vi "TDMS Write Group Data.vi"(8 "error in (no error)":errorcluster, 9 "Fields Array":T1[](array[typedef]), 10 "Channel Group":string, 11 "TDMS File Ref":refnum<k34>) -> (0 "error out":errorcluster, 3 "TDMS File Ref":refnum<k34>, 4 "Execution Time (ms)":u32)   [LabVIEW 2011]
uses:
  database/Fields/Field Record.ctl
  database/Fields/Field DataTypes.ctl
  database/Fields/Field NextItem.ctl
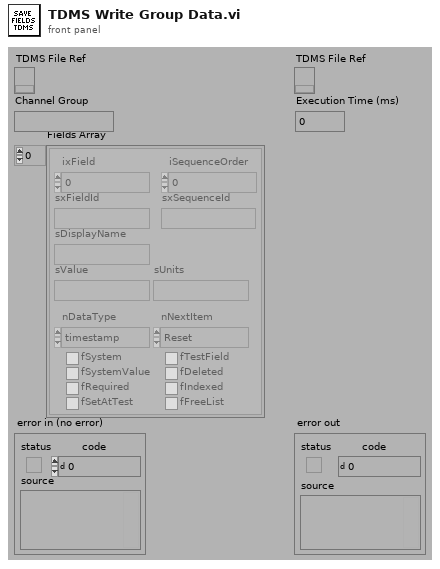
[diagram p1: front panel]
types:
  T1 = typedef "Field Record.ctl" = cluster{"ixField":i32, "iSequenceOrder":i32, "sxFieldId":string, "sxSequenceId":string, "sDisplayName":string, "sValue":string, "sUnits":string, "nDataType":T2, "nNextItem":T3, "fSystem":bool, "fSystemValue":bool, "fRequired":bool, "fSetAtTest":bool, "fTestField":bool, "fDeleted":bool, "fIndexed":bool, "fFreeList":bool}
  T2 = typedef "Field DataTypes.ctl" = enum32{"text", "numeric", "list", "timestamp", "boolean"}
  T3 = typedef "Field NextItem.ctl" = enum32{"Reset", "Retain", "Auto-Increment"}
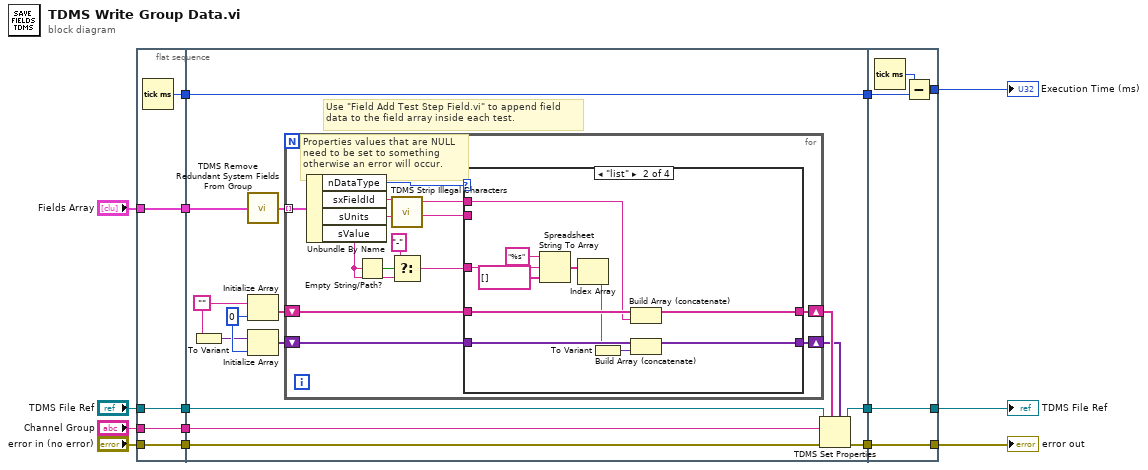
[diagram p0: block diagram]
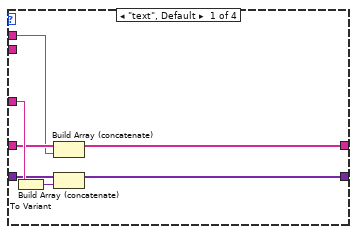
[diagram p2: hidden frame]
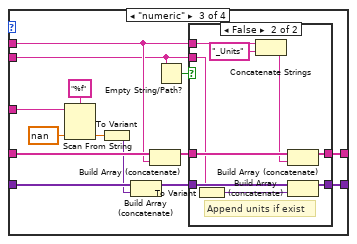
[diagram p3: hidden frame]
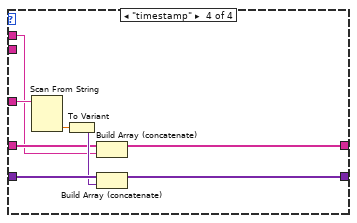
[diagram p5: hidden frame]
diagram:
  n1 = flat-sequence {
    tunnel: "Channel Group" -> [w17]
    tunnel: "error in (no error)" -> [w18]
    tunnel: "TDMS File Ref" -> [w19]
    tunnel: "Fields Array" -> [w20]
    tunnel: [w20] -> w7
    tunnel: [w19] -> w6
    tunnel: [w18] -> w5
    tunnel: [w17] -> w4
    tunnel: [w16] -> w2
    tunnel: [w30] -> w9
    tunnel: [w33] -> w8
    tunnel: w7 -> [w22]
    tunnel: w6 -> [w35]
    tunnel: w5 -> [w34]
    tunnel: w4 -> [w32]
    tunnel: [w31] -> w3
    tunnel: w2 -> [w31]
    tunnel: [w103] -> w11
    tunnel: [w104] -> w14
    tunnel: w9 -> [w104]
    tunnel: w8 -> [w103]
    tunnel: w3 -> [w101]
    tunnel: [w100] -> w1
    frame #0 {
      n2 = Tick Count (ms)() -> (millisecond timer value=w16:u32)
    }
    frame #1 {
      w27 = 0 ("dimension size")
      w23 = ""
      # "Use \"Field Add Test Step Field.vi\" to append field\ndata to the field array inside each test."
      n3 = To Variant(anything=w23) -> (Variant=w26:variant)
      n4 = call "TDMS Remove Redundant System Fields From Group.vi"("Fields In"=w22) -> ("Fields Out"=w21:T1[])
      n5 = Initialize Array(w23, w27) -> (w29:string[])
      n6 = Initialize Array(w26, w27) -> (w28:variant[])
      n7 = for {
        tunnel: w21 -> [w48] mode=indexing
        shift-right: [w40] -> w25
        shift-left: w29 -> [w42]
        shift-right: [w41] -> w24
        shift-left: w28 -> [w43]
        # "Properties values that are NULL\nneed to be set to something\notherwise an error will occur."
        n8 = Unbundle By Name(w48) -> ("nDataType"=w38:T2, "sxFieldId"=w44:string, "sUnits"=w36:string, "sValue"=w37:string)
        n9 = Empty String/Path?(string/path=w37) -> (empty?=w47:bool)
        n10 = call "TDMS Strip Illegal Characters.vi"("String"=w44) -> ("Legal String"=w39:string)  [unwired: 4 out]
        n11 = Select(t="-", s=w47, f=w37) -> (s? t:f=w46:string)
        n12 = case shown="\"numeric\"" w38 {
          tunnel: w46 -> [w55 w60 w75 w98]
          tunnel: w43 -> [w52 w64 w79 w97]
          tunnel: w42 -> [w54 w66 w80 w94]
          tunnel: [w49 w61 w70 w95] -> w41
          tunnel: [w53 w65 w71 w93] -> w40
          tunnel: w39 -> [w50 w62 w69 w92]
          tunnel: w36 -> [_ _ w67 _]
          frame "text", Default {
            n13 = To Variant(anything=w55) -> (Variant=w51:variant)
            n14 = Build Array (concatenate)(w54, w50) -> (w53:string[])
            n15 = Build Array (concatenate)(w52, w51) -> (w49:variant[])
          }
          frame "list" {
            n16 = Spreadsheet String To Array(format string="%s" ("delimiter (Tab)"), spreadsheet string=w60, array type (2D Dbl)=string[] []) -> (array=w58:string[])  [unwired: 1 in]
            n17 = Index Array(array=w58) -> (element=w57:string)  [unwired: 1 in]
            n18 = To Variant(anything=w57) -> (Variant=w63:variant)
            n19 = Build Array (concatenate)(w66, w62) -> (w65:string[])
            n20 = Build Array (concatenate)(w64, w63) -> (w61:variant[])
          }
          frame "numeric" {
            n21 = Scan From String(format string="%f", input string=w75, default 1=nan) -> (output 1=w77:dbl)  [unwired: 2 in, 3 out]
            n22 = To Variant(anything=w77) -> (Variant=w78:variant)
            n23 = Build Array (concatenate)(w79, w78) -> (w72:variant[])
            n24 = Build Array (concatenate)(w80, w69) -> (w73:string[])
            n25 = Empty String/Path?(string/path=w67) -> (empty?=w68:bool)
            n26 = case shown="True" w68 {
              tunnel: w73 -> [w82 w91]
              tunnel: w72 -> [w81 w90]
              tunnel: [w82 w89] -> w71
              tunnel: [w81 w88] -> w70
              tunnel: w69 -> [_ w86]
              tunnel: w67 -> [_ w83]
              frame True {
              }
              frame False {
                # "Append units if exist"
                n27 = To Variant(anything=w83) -> (Variant=w84:variant)
                n28 = Concatenate Strings(w86, "_Units") -> (w85:string)
                n29 = Build Array (concatenate)(w91, w85) -> (w89:string[])
                n30 = Build Array (concatenate)(w90, w84) -> (w88:variant[])
              }
            }
          }
          frame "timestamp" {
            n31 = Scan From String(input string=w98) -> (output 1=w99:dbl)  [unwired: 3 in, 4 out]
            n32 = To Variant(anything=w99) -> (Variant=w96:variant)
            n33 = Build Array (concatenate)(w94, w92) -> (w93:string[])
            n34 = Build Array (concatenate)(w97, w96) -> (w95:variant[])
          }
        }
      }
      n35 = TDMS Set Properties(5:w24, 7:w25, 8:w34, 10:w32, 11:w35) -> (0:w30:errorcluster, 3:w33:refnum<k34>)  [unwired: 3 out]
    }
    frame #2 {
      n36 = Tick Count (ms)() -> (millisecond timer value=w102:u32)
      n37 = Subtract(x=w102, y=w101) -> (x-y=w100:u32)
    }
  }
  "error out" <- w14
  "TDMS File Ref" <- w11
  "Execution Time (ms)" <- w1
